vi "HDI Pat Match Full with Move BL.vi"(5 "controller in":refnum<k24>, 11 "error in":errorcluster) -> (4 "In Range?":bool, 8 "x rel move":dbl, 10 "y rel move":dbl, 15 "error out":errorcluster)   [LabVIEW 2011]
uses:
  C:/Users/Admin/Desktop/Gantry Code Transfer/source/Code Transfer/Aerotech.A3200.dll
  Aerotech.A3200.dll
  <vilib>/vision/driver/NI_Vision_Acquisition_Software.lvlib
panel:
  out "Angle Between Lines":dbl
  out "Diagnostic Log":string
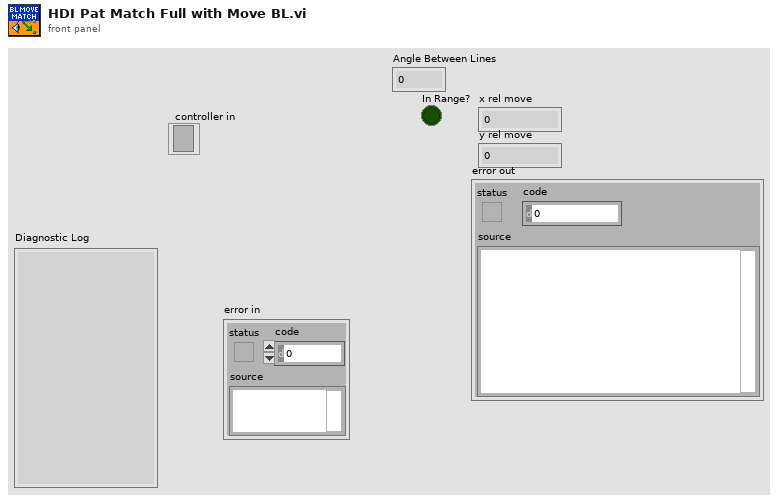
[diagram p1: front panel]
types:
  T1 = typedef "IMAQdx.ctl" = refnum<k21>
  T2 = typedef "IMAQ Image.ctl" = refnum<image>
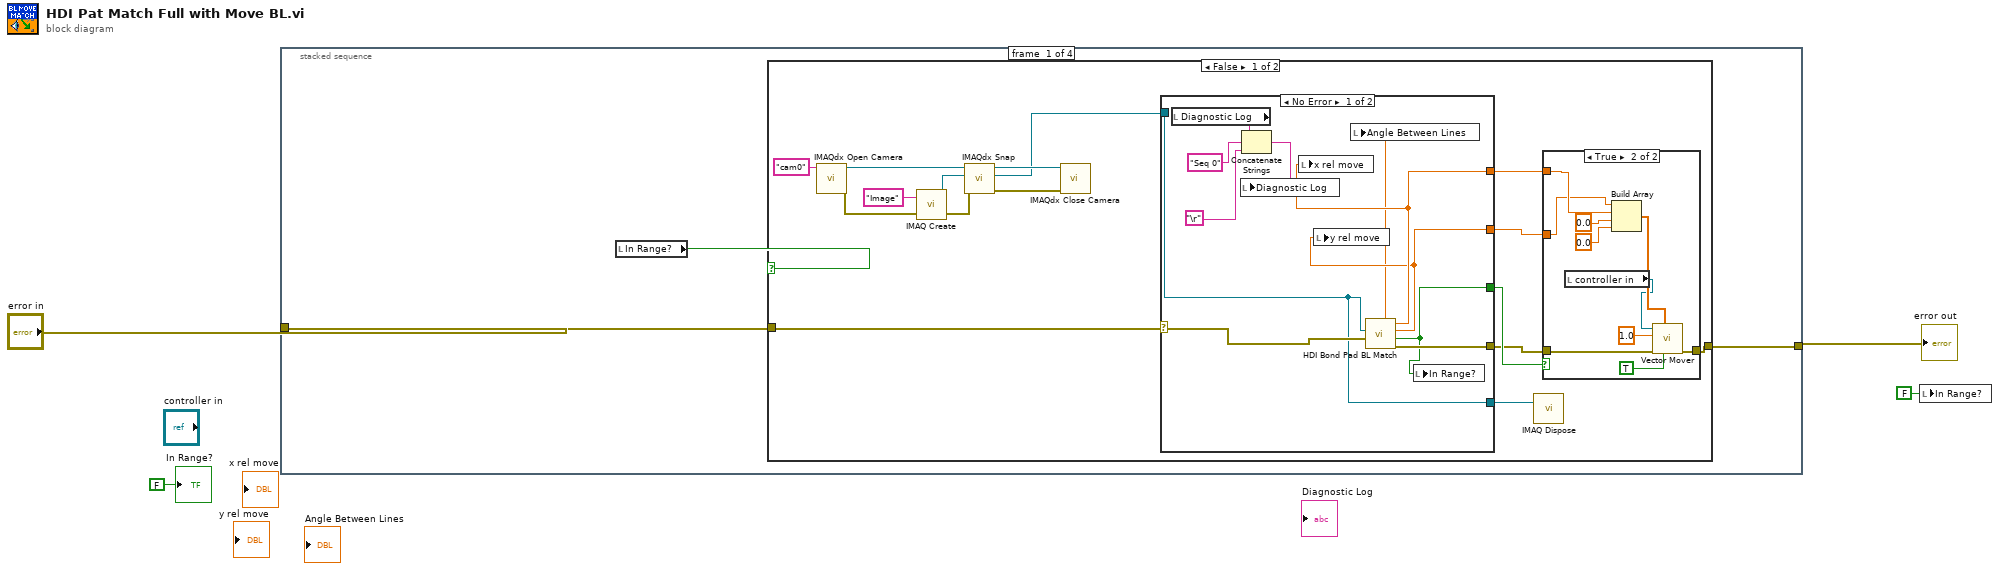
[diagram p0: block diagram]
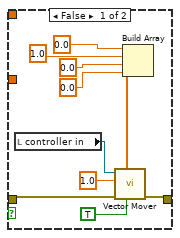
[diagram p2: hidden frame]
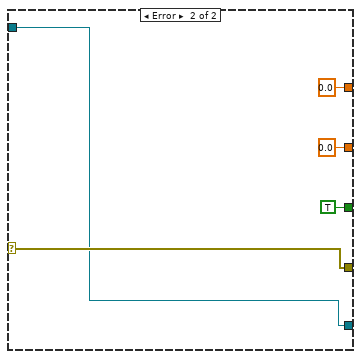
[diagram p3: hidden frame]
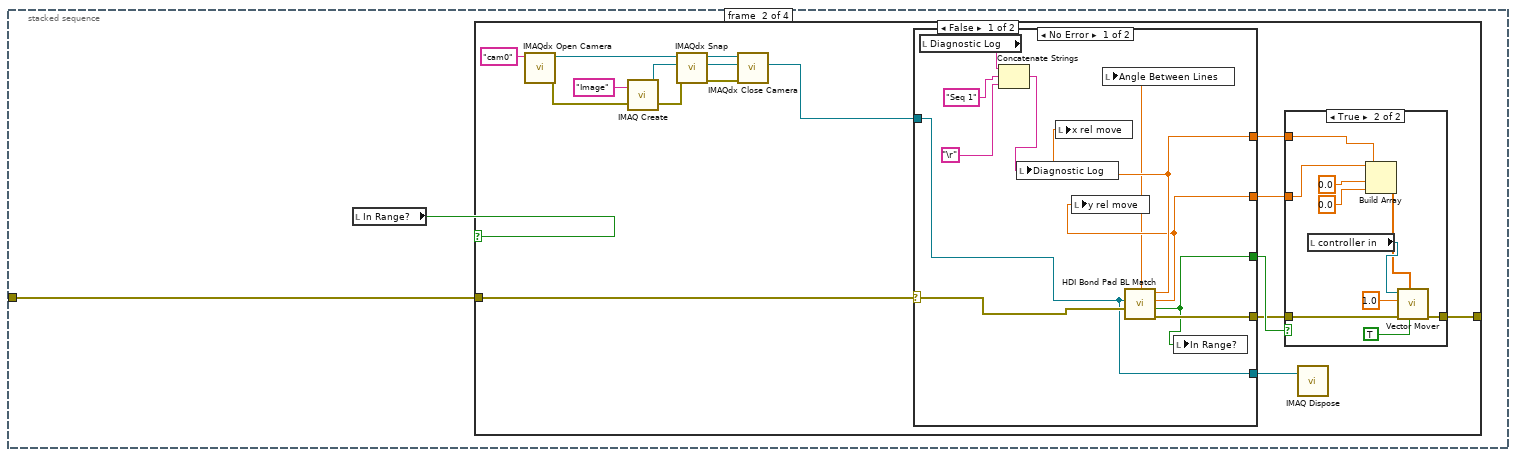
[diagram p5: hidden frame]
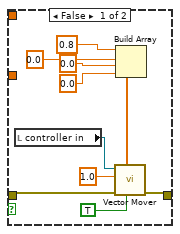
[diagram p6: hidden frame]
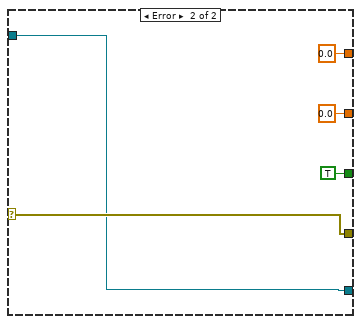
[diagram p7: hidden frame]
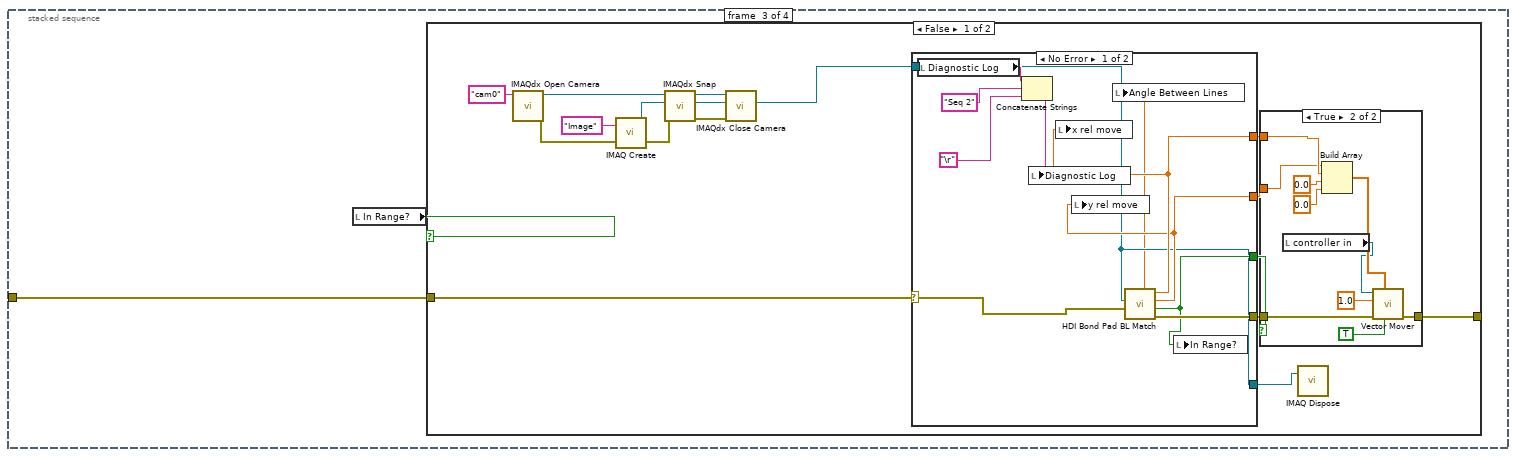
[diagram p9: hidden frame]
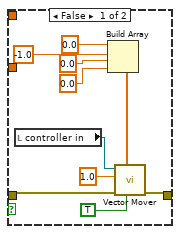
[diagram p10: hidden frame]
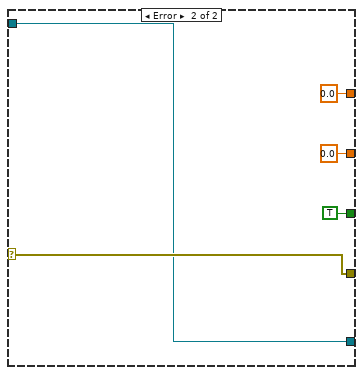
[diagram p11: hidden frame]
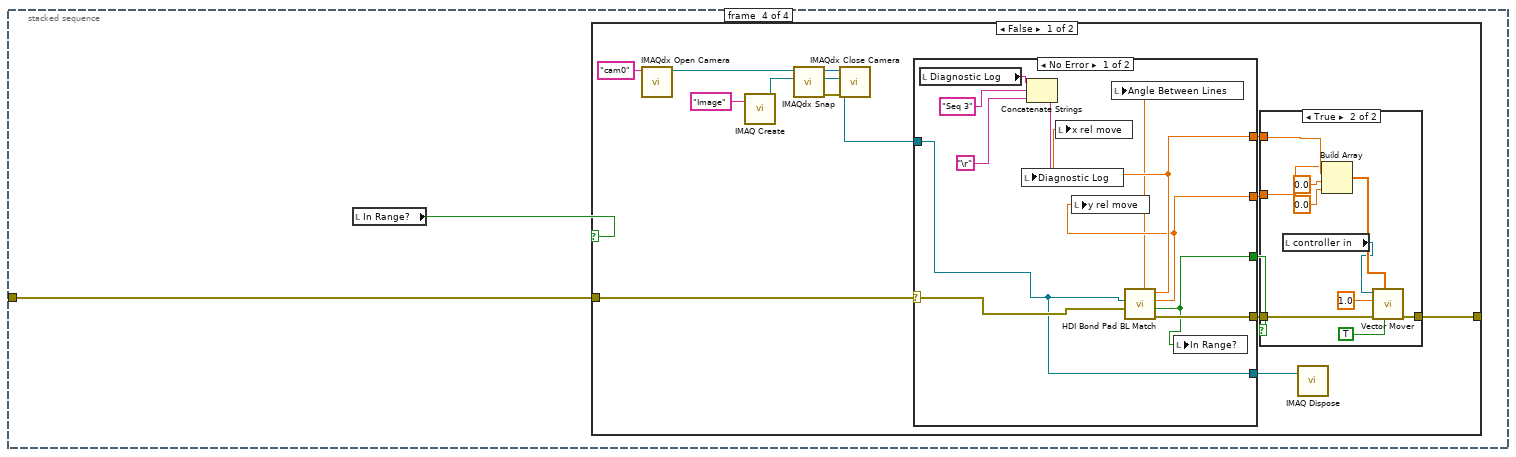
[diagram p13: hidden frame]
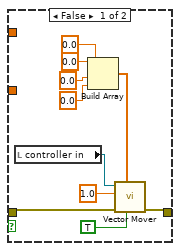
[diagram p14: hidden frame]
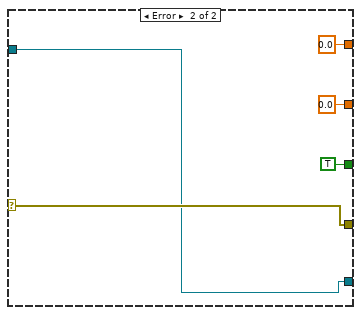
[diagram p15: hidden frame]
diagram:
  n1 = stacked-sequence {
    tunnel: "error in" -> [w7 w62 w117 w172]
    tunnel: [w6 _ _ _] -> w4
    frame #0 {
      n2 = local read "In Range?"() -> (w5:bool)
      n3 = case shown="False" w5 {
        tunnel: w7 -> [w23 w60]
        tunnel: [w20 w60] -> w6
        frame False {
          n4 = call <vilib>:"IMAQdx Open Camera.vi"("Session In"="cam0" ("Interface Name")) -> ("error out"=w14:errorcluster, "Session Out"=w9:T1)  [unwired: 9 in]
          n5 = call "IMAQ Create"("Image Name"="Image", "error in (no error)"=w14) -> ("New Image"=w11:T2, "error out"=w10:errorcluster)  [unwired: 3 in]
          n6 = call <vilib>:"IMAQdx Snap.vi"("error in"=w10, "Image In"=w11, "Session In"=w9) -> ("error out"=w12:errorcluster, "Image Out"=w8:T2, "Session Out"=w13:T1)  [unwired: 6 in]
          n7 = call <vilib>:"IMAQdx Close Camera.vi"("error in"=w12, "Session In"=w13) -> ()  [unwired: 9 in, 1 out]
          n8 = case shown="No Error" w23 {
            selector: w23 -> [w53 w59]
            tunnel: [w54 w59] -> w21
            tunnel: [w50 TRUE ("Matched?")] -> w22
            tunnel: [w52 0.0 ("x rel move")] -> w19
            tunnel: [w51 0.0 ("y rel move")] -> w18
            tunnel: w8 -> [w45 w55]
            tunnel: [w45 w55] -> w17
            frame No Error {
              n9 = local read "Diagnostic Log"() -> (w46:string)
              n10 = Concatenate Strings(w46, "Seq 0", "\r") -> (w49:string)
              n11 = local write "Diagnostic Log"(w49) -> ()
              n12 = call "HDI Bond Pad BL Match.vi"("error in (no error)"=w53, "Image Src"=w45) -> ("error out"=w54:errorcluster, "In Range?"=w50:bool, "y rel move"=w51:dbl, "x rel move"=w52:dbl, "Angle Between Lines"=w44:dbl)  [unwired: 5 in]
              n13 = local write "x rel move"(w52) -> ()
              n14 = local write "y rel move"(w51) -> ()
              n15 = local write "Angle Between Lines"(w44) -> ()
              n16 = local write "In Range?"(w50) -> ()
            }
            frame Error {
            }
          }
          n17 = call "IMAQ Dispose"("Image"=w17) -> ()  [unwired: 5 in, 1 out]
          n18 = case shown="True" w22 {
            tunnel: w21 -> [w31 w43]
            tunnel: [w26 w42] -> w20
            tunnel: w19 -> [_ w35]
            tunnel: w18 -> [_ w34]
            frame False {
              n19 = local read "controller in"() -> (w25:refnum<k24>)
              n20 = Build Array(0.0 ("element"), 1.0 ("element"), 0.0 ("element"), 0.0 ("element")) -> (w28:dbl[])
              n21 = call "Vector Mover.vi"("Absolute/Relative (F/T)"=TRUE, "Movement Vector"=w28, "error in (no error)"=w31, "Vector Speed"=1.0, "controller in"=w25) -> ("error out"=w26:errorcluster)  [unwired: 1 in, 3 out]
            }
            frame True {
              n22 = local read "controller in"() -> (w36:refnum<k24>)
              n23 = Build Array(w34, w35, 0.0 ("element"), 0.0 ("element")) -> (w37:dbl[])
              n24 = call "Vector Mover.vi"("Absolute/Relative (F/T)"=TRUE, "Movement Vector"=w37, "error in (no error)"=w43, "Vector Speed"=1.0, "controller in"=w36) -> ("error out"=w42:errorcluster)  [unwired: 1 in, 3 out]
            }
          }
        }
        frame True {
        }
      }
    }
    frame #1 {
      n25 = local read "In Range?"() -> (w61:bool)
      n26 = case shown="False" w61 {
        tunnel: w62 -> [w78 w115]
        tunnel: [w75 w115] -> _
        frame False {
          n27 = call <vilib>:"IMAQdx Open Camera.vi"("Session In"="cam0" ("Interface Name")) -> ("error out"=w69:errorcluster, "Session Out"=w64:T1)  [unwired: 9 in]
          n28 = call "IMAQ Create"("Image Name"="Image", "error in (no error)"=w69) -> ("New Image"=w66:T2, "error out"=w65:errorcluster)  [unwired: 3 in]
          n29 = call <vilib>:"IMAQdx Snap.vi"("error in"=w65, "Image In"=w66, "Session In"=w64) -> ("error out"=w67:errorcluster, "Image Out"=w63:T2, "Session Out"=w68:T1)  [unwired: 6 in]
          n30 = call <vilib>:"IMAQdx Close Camera.vi"("error in"=w67, "Session In"=w68) -> ()  [unwired: 9 in, 1 out]
          n31 = case shown="No Error" w78 {
            selector: w78 -> [w108 w114]
            tunnel: [w109 w114] -> w76
            tunnel: [w105 TRUE ("Matched?")] -> w77
            tunnel: [w107 0.0 ("x rel move")] -> w74
            tunnel: [w106 0.0 ("y rel move")] -> w73
            tunnel: w63 -> [w100 w110]
            tunnel: [w100 w110] -> w72
            frame No Error {
              n32 = local read "Diagnostic Log"() -> (w101:string)
              n33 = Concatenate Strings(w101, "Seq 1", "\r") -> (w104:string)
              n34 = local write "Diagnostic Log"(w104) -> ()
              n35 = call "HDI Bond Pad BL Match.vi"("error in (no error)"=w108, "Image Src"=w100) -> ("error out"=w109:errorcluster, "In Range?"=w105:bool, "y rel move"=w106:dbl, "x rel move"=w107:dbl, "Angle Between Lines"=w99:dbl)  [unwired: 5 in]
              n36 = local write "x rel move"(w107) -> ()
              n37 = local write "y rel move"(w106) -> ()
              n38 = local write "Angle Between Lines"(w99) -> ()
              n39 = local write "In Range?"(w105) -> ()
            }
            frame Error {
            }
          }
          n40 = case shown="True" w77 {
            tunnel: w76 -> [w86 w98]
            tunnel: [w80 w97] -> w75
            tunnel: w74 -> [_ w90]
            tunnel: w73 -> [_ w89]
            frame False {
              n41 = local read "controller in"() -> (w79:refnum<k24>)
              n42 = Build Array(0.8 ("element"), 0.0 ("element"), 0.0 ("element"), 0.0 ("element")) -> (w83:dbl[])
              n43 = call "Vector Mover.vi"("Absolute/Relative (F/T)"=TRUE, "Movement Vector"=w83, "error in (no error)"=w86, "Vector Speed"=1.0, "controller in"=w79) -> ("error out"=w80:errorcluster)  [unwired: 1 in, 3 out]
            }
            frame True {
              n44 = local read "controller in"() -> (w92:refnum<k24>)
              n45 = Build Array(w89, w90, 0.0 ("element"), 0.0 ("element")) -> (w91:dbl[])
              n46 = call "Vector Mover.vi"("Absolute/Relative (F/T)"=TRUE, "Movement Vector"=w91, "error in (no error)"=w98, "Vector Speed"=1.0, "controller in"=w92) -> ("error out"=w97:errorcluster)  [unwired: 1 in, 3 out]
            }
          }
          n47 = call "IMAQ Dispose"("Image"=w72) -> ()  [unwired: 5 in, 1 out]
        }
        frame True {
        }
      }
    }
    frame #2 {
      n48 = local read "In Range?"() -> (w116:bool)
      n49 = case shown="False" w116 {
        tunnel: w117 -> [w133 w170]
        tunnel: [w130 w170] -> _
        frame False {
          n50 = call <vilib>:"IMAQdx Open Camera.vi"("Session In"="cam0" ("Interface Name")) -> ("error out"=w124:errorcluster, "Session Out"=w119:T1)  [unwired: 9 in]
          n51 = call "IMAQ Create"("Image Name"="Image", "error in (no error)"=w124) -> ("New Image"=w121:T2, "error out"=w120:errorcluster)  [unwired: 3 in]
          n52 = call <vilib>:"IMAQdx Snap.vi"("error in"=w120, "Image In"=w121, "Session In"=w119) -> ("error out"=w122:errorcluster, "Image Out"=w118:T2, "Session Out"=w123:T1)  [unwired: 6 in]
          n53 = call <vilib>:"IMAQdx Close Camera.vi"("error in"=w122, "Session In"=w123) -> ()  [unwired: 9 in, 1 out]
          n54 = case shown="No Error" w133 {
            selector: w133 -> [w163 w169]
            tunnel: [w164 w169] -> w131
            tunnel: [w160 TRUE ("Matched?")] -> w132
            tunnel: [w162 0.0 ("x rel move")] -> w129
            tunnel: [w161 0.0 ("y rel move")] -> w128
            tunnel: w118 -> [w155 w165]
            tunnel: [w155 w165] -> w127
            frame No Error {
              n55 = local read "Diagnostic Log"() -> (w156:string)
              n56 = Concatenate Strings(w156, "Seq 2", "\r") -> (w159:string)
              n57 = local write "Diagnostic Log"(w159) -> ()
              n58 = call "HDI Bond Pad BL Match.vi"("error in (no error)"=w163, "Image Src"=w155) -> ("error out"=w164:errorcluster, "In Range?"=w160:bool, "y rel move"=w161:dbl, "x rel move"=w162:dbl, "Angle Between Lines"=w154:dbl)  [unwired: 5 in]
              n59 = local write "x rel move"(w162) -> ()
              n60 = local write "y rel move"(w161) -> ()
              n61 = local write "Angle Between Lines"(w154) -> ()
              n62 = local write "In Range?"(w160) -> ()
            }
            frame Error {
            }
          }
          n63 = case shown="True" w132 {
            tunnel: w131 -> [w141 w153]
            tunnel: [w135 w152] -> w130
            tunnel: w129 -> [_ w145]
            tunnel: w128 -> [_ w144]
            frame False {
              n64 = local read "controller in"() -> (w134:refnum<k24>)
              n65 = Build Array(0.0 ("element"), -1.0 ("element"), 0.0 ("element"), 0.0 ("element")) -> (w138:dbl[])
              n66 = call "Vector Mover.vi"("Absolute/Relative (F/T)"=TRUE, "Movement Vector"=w138, "error in (no error)"=w141, "Vector Speed"=1.0, "controller in"=w134) -> ("error out"=w135:errorcluster)  [unwired: 1 in, 3 out]
            }
            frame True {
              n67 = local read "controller in"() -> (w146:refnum<k24>)
              n68 = Build Array(w144, w145, 0.0 ("element"), 0.0 ("element")) -> (w147:dbl[])
              n69 = call "Vector Mover.vi"("Absolute/Relative (F/T)"=TRUE, "Movement Vector"=w147, "error in (no error)"=w153, "Vector Speed"=1.0, "controller in"=w146) -> ("error out"=w152:errorcluster)  [unwired: 1 in, 3 out]
            }
          }
          n70 = call "IMAQ Dispose"("Image"=w127) -> ()  [unwired: 5 in, 1 out]
        }
        frame True {
        }
      }
    }
    frame #3 {
      n71 = local read "In Range?"() -> (w171:bool)
      n72 = case shown="False" w171 {
        tunnel: w172 -> [w186 w223]
        tunnel: [w183 w223] -> _
        frame False {
          n73 = call <vilib>:"IMAQdx Open Camera.vi"("Session In"="cam0" ("Interface Name")) -> ("Session Out"=w174:T1)  [unwired: 9 in, 1 out]
          n74 = call "IMAQ Create"("Image Name"="Image") -> ("New Image"=w175:T2)  [unwired: 4 in, 1 out]
          n75 = call <vilib>:"IMAQdx Snap.vi"("Image In"=w175, "Session In"=w174) -> ("error out"=w176:errorcluster, "Image Out"=w173:T2, "Session Out"=w177:T1)  [unwired: 7 in]
          n76 = call <vilib>:"IMAQdx Close Camera.vi"("error in"=w176, "Session In"=w177) -> ()  [unwired: 9 in, 1 out]
          n77 = case shown="No Error" w186 {
            selector: w186 -> [w216 w222]
            tunnel: [w217 w222] -> w184
            tunnel: [w213 TRUE ("Matched?")] -> w185
            tunnel: [w215 0.0 ("x rel move")] -> w182
            tunnel: [w214 0.0 ("y rel move")] -> w181
            tunnel: w173 -> [w208 w218]
            tunnel: [w208 w218] -> w180
            frame No Error {
              n78 = local read "Diagnostic Log"() -> (w209:string)
              n79 = Concatenate Strings(w209, "Seq 3", "\r") -> (w212:string)
              n80 = local write "Diagnostic Log"(w212) -> ()
              n81 = call "HDI Bond Pad BL Match.vi"("error in (no error)"=w216, "Image Src"=w208) -> ("error out"=w217:errorcluster, "In Range?"=w213:bool, "y rel move"=w214:dbl, "x rel move"=w215:dbl, "Angle Between Lines"=w207:dbl)  [unwired: 5 in]
              n82 = local write "x rel move"(w215) -> ()
              n83 = local write "y rel move"(w214) -> ()
              n84 = local write "Angle Between Lines"(w207) -> ()
              n85 = local write "In Range?"(w213) -> ()
            }
            frame Error {
            }
          }
          n86 = case shown="True" w185 {
            tunnel: w184 -> [w194 w206]
            tunnel: [w188 w205] -> w183
            tunnel: w182 -> [_ w198]
            tunnel: w181 -> [_ w197]
            frame False {
              n87 = local read "controller in"() -> (w187:refnum<k24>)
              n88 = Build Array(0.0 ("element"), 0.0 ("element"), 0.0 ("element"), 0.0 ("element")) -> (w191:dbl[])
              n89 = call "Vector Mover.vi"("Absolute/Relative (F/T)"=TRUE, "Movement Vector"=w191, "error in (no error)"=w194, "Vector Speed"=1.0, "controller in"=w187) -> ("error out"=w188:errorcluster)  [unwired: 1 in, 3 out]
            }
            frame True {
              n90 = local read "controller in"() -> (w199:refnum<k24>)
              n91 = Build Array(w197, w198, 0.0 ("element"), 0.0 ("element")) -> (w200:dbl[])
              n92 = call "Vector Mover.vi"("Absolute/Relative (F/T)"=TRUE, "Movement Vector"=w200, "error in (no error)"=w206, "Vector Speed"=1.0, "controller in"=w199) -> ("error out"=w205:errorcluster)  [unwired: 1 in, 3 out]
            }
          }
          n93 = call "IMAQ Dispose"("Image"=w180) -> ()  [unwired: 5 in, 1 out]
        }
        frame True {
        }
      }
    }
  }
  "error out" <- w4
  n94 = local write "In Range?"(FALSE ("In Range?")) -> ()
  "In Range?" <- FALSE ("In Range?")
